vi "Laser_Setup_Options.vi"() -> (0 "Lasers IP Numbers":string[](array[string]), 1 "Wavelengths":dbl[](array[numeric]), 2 "error out":errorcluster, 3 "Lasers":string[](array[string]))   [LabVIEW 2022 SP3]
uses:
  <vilib>/Utility/error.llb/Trim Whitespace One-Sided.vi
  Globals/LDA_global.vi
  Globals/Constants_global.vi
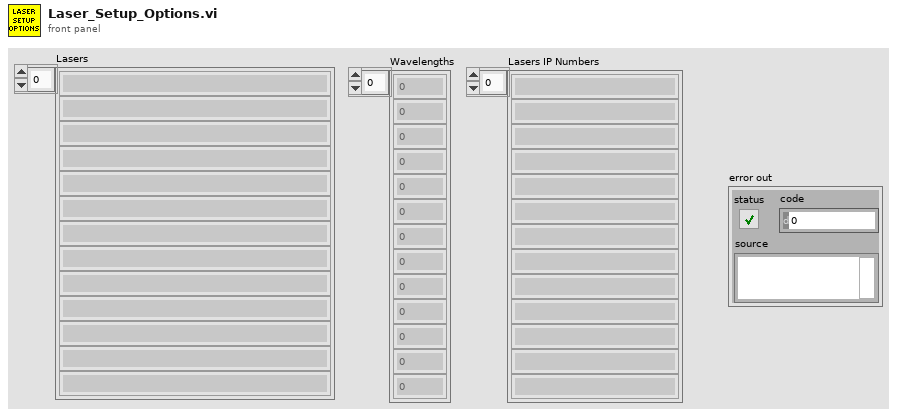
[diagram p1: front panel]
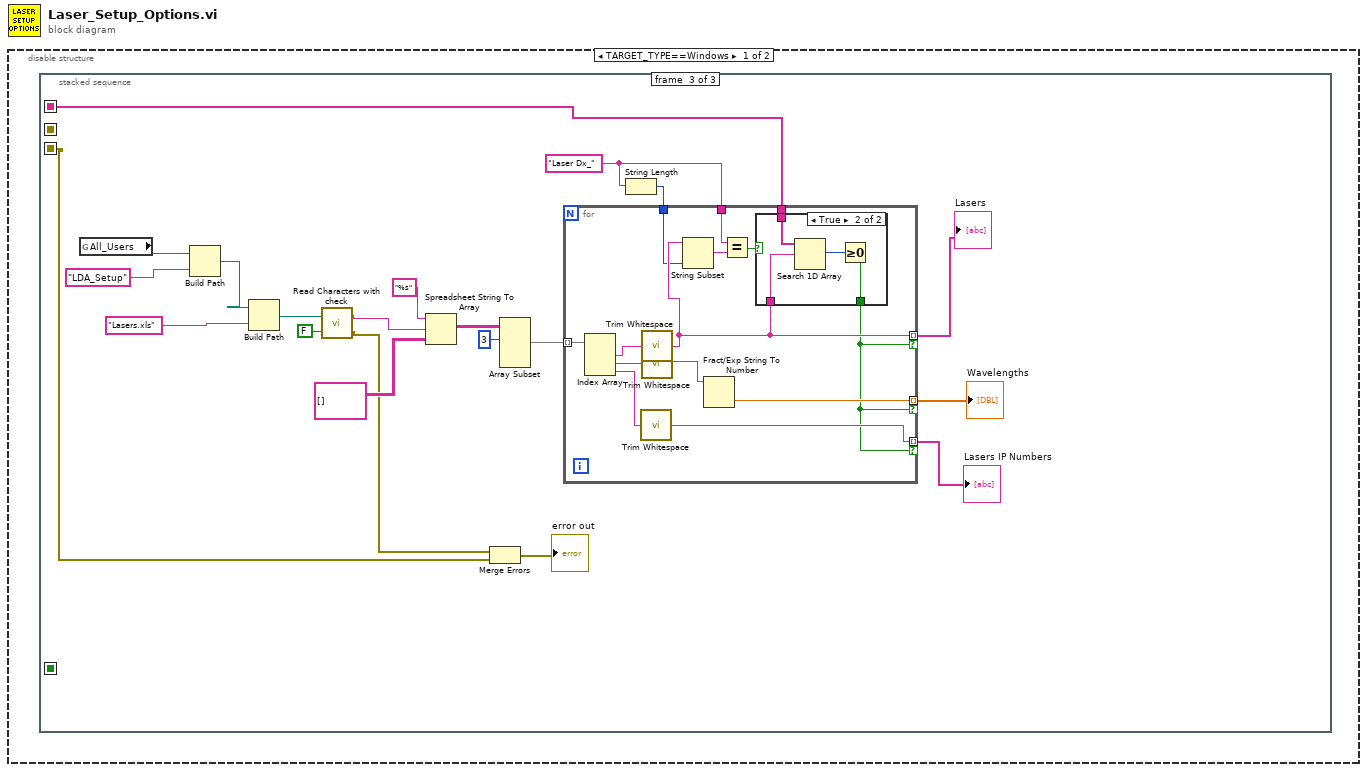
[diagram p0: block diagram]
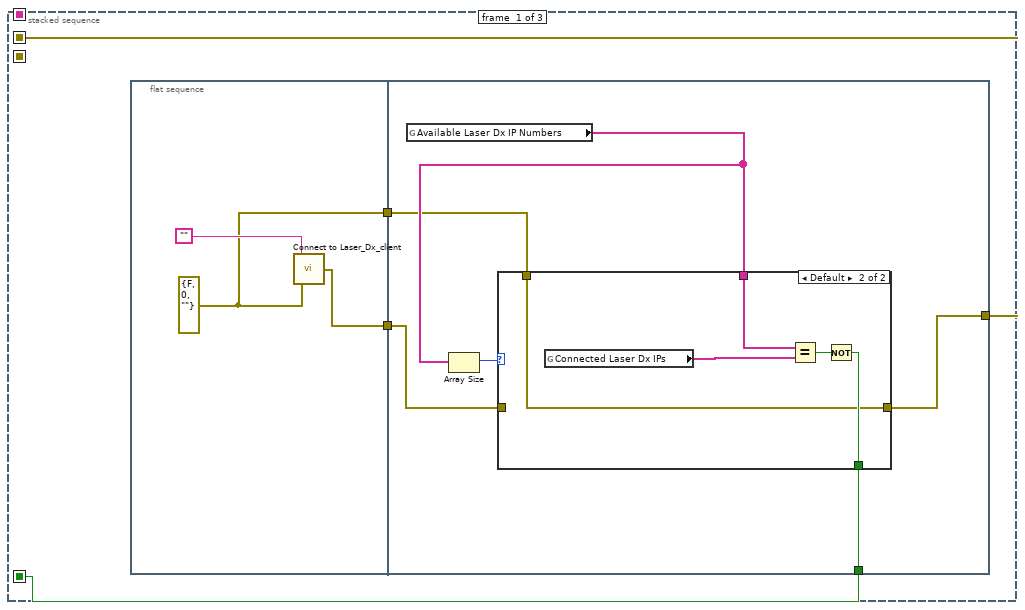
[diagram p2: hidden frame]
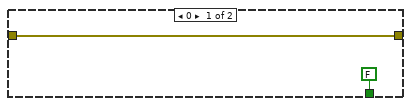
[diagram p3: hidden frame]
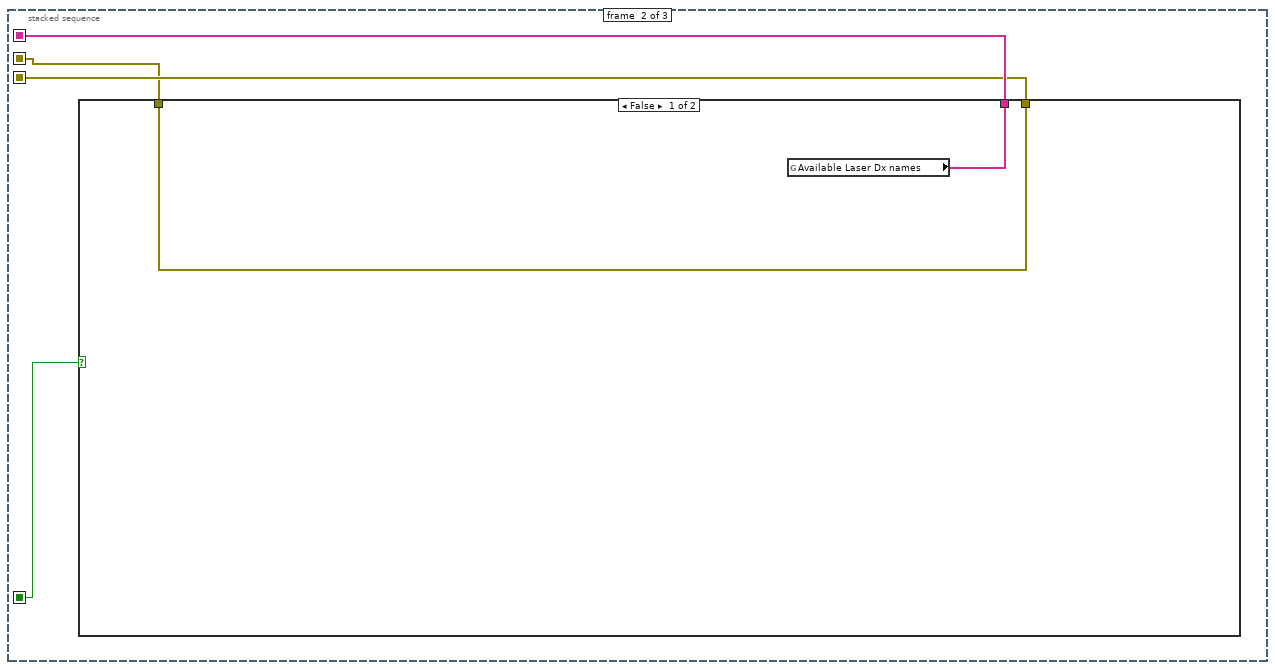
[diagram p4: hidden frame]
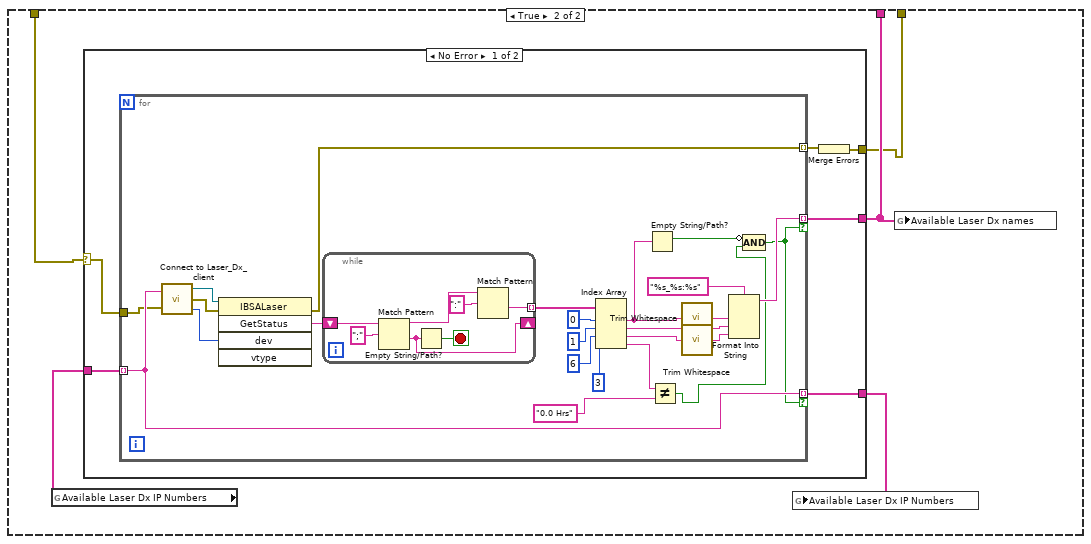
[diagram p5: hidden frame]
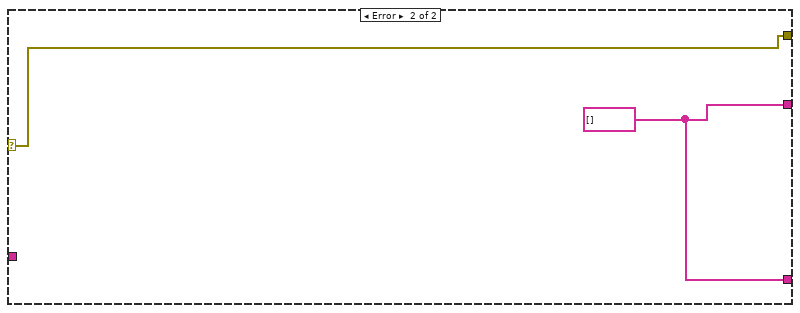
[diagram p6: hidden frame]
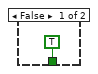
[diagram p7: hidden frame]
diagram:
  n1 = disable-structure shown="TARGET_TYPE==Windows" {
    frame condition #0 (active) {
      n2 = stacked-sequence {
        seq-local: [_ w24 _] -> [_ _ w77]
        seq-local: [_ w23 _] -> [_ _ w76]
        seq-local: [w3 _ _] -> [_ w22 _]
        seq-local: [w1 _ _] -> [_ w21 _]
        frame #0 {
          n3 = flat-sequence {
            tunnel: [w6] -> w4
            tunnel: [w5] -> w2
            tunnel: w4 -> [w10]
            tunnel: [w11] -> w3
            tunnel: w2 -> [w8]
            tunnel: [w9] -> w1
            frame #0 {
              w5 = errorcluster {"status"=FALSE, "code"=0, "source"=""} ("error in (no error)")
              n4 = call "Connect to Laser_Dx_client.vi"("Laser IP Number"="", "error in (no error)"=w5) -> ("error out"=w6:errorcluster)  [unwired: 2 out]
            }
            frame #1 {
              n5 = global read "LDA_global.vi" "Available Laser Dx IP Numbers"() -> (w13:string[])
              n6 = Array Size(array=w13) -> (size(s)=w12:i32)
              n7 = case shown="Default" w12 {
                tunnel: w13 -> [_ w19]
                tunnel: [w15 w16] -> w11
                tunnel: w10 -> [w15 _]
                tunnel: [FALSE w17] -> w9
                tunnel: w8 -> [_ w16]
                frame 0 {
                }
                frame Default {
                  n8 = global read "LDA_global.vi" "Connected Laser Dx IPs"() -> (w20:string[])
                  n9 = Equal?(x=w19, y=w20) -> (x = y?=w18:bool)
                  n10 = Not(x=w18) -> (.not. x?=w17:bool)
                }
              }
            }
          }
        }
        frame #1 {
          n11 = case shown="False" w21 {
            tunnel: [w26 w30] -> w24
            tunnel: [w25 w28] -> w23
            tunnel: w22 -> [w25 w27]
            frame False {
              n12 = global read "LDA_global.vi" "Available Laser Dx names"() -> (w26:string[])
            }
            frame True {
              n13 = global read "LDA_global.vi" "Available Laser Dx IP Numbers"() -> (w31:string[])
              n14 = case shown="No Error" w27 {
                selector: w27 -> [w32 w70]
                tunnel: w31 -> [w37 _]
                tunnel: [w36 w69] -> w30
                tunnel: [w35 w69] -> w29
                tunnel: [w33 w70] -> w28
                frame No Error {
                  n15 = for {
                    tunnel: [w51] -> w36 mode=indexing if=w38
                    tunnel: w37 -> [w46] mode=indexing
                    tunnel: [w46] -> w35 mode=indexing if=w38
                    tunnel: w32 -> [w43]
                    tunnel: [w42] -> w34 mode=indexing
                    n16 = call "Connect to Laser_Dx_client.vi"("Laser IP Number"=w46, "error in (no error)"=w43) -> ("Laser_Dx"=w50:refnum<k7>, "error out"=w45:errorcluster, "Channel"=w44:i64)
                    n17 = invoke class="IBSALaser" method="GetStatus"(reference=w50, error in=w45, "dev"=w44) -> (error out=w42:errorcluster, "GetStatus"=w52:string)  [unwired: 2 in, 3 out]
                    n18 = while {
                      shift-right: [w65] -> _
                      shift-left: w52 -> [w67]
                      tunnel: [w62] -> w58 mode=indexing
                      stop <- w66 stop-if-true
                      n19 = Match Pattern(string=w67, regular expression=";") -> (before substring=w64:string, after substring=w65:string)  [unwired: 1 in, 2 out]
                      n20 = Empty String/Path?(string/path=w65) -> (empty?=w66:bool)
                      n21 = Match Pattern(string=w64, regular expression=":") -> (after substring=w62:string)  [unwired: 1 in, 3 out]
                    }
                    n22 = Index Array(array=w58, index #1=0 ("index"), index #2=1 ("index"), index #3=6 ("index"), index #4=3 ("index")) -> (element #1=w41:string, element #2=w56:string, element #3=w59:string, element #4=w47:string)
                    n23 = Empty String/Path?(string/path=w41) -> (empty?=w40:bool)
                    n24 = Not Equal?(x=w47, y="0.0 Hrs" ("element")) -> (x != y?=w39:bool)
                    n25 = call <vilib>:"Trim Whitespace.vi"("string"=w41) -> ("trimmed string"=w61:string)  [unwired: 1 in]
                    n26 = call <vilib>:"Trim Whitespace.vi"("string"=w59) -> ("trimmed string"=w60:string)  [unwired: 1 in]
                    n27 = Format Into String(format string="%s_%s:%s", w61, w56, w60) -> (resulting string=w51:string)  [unwired: 2 in, 1 out]
                    n28 = Compound Arithmetic op=AND(invert w40, w39) -> (w38:bool)
                  }
                  n29 = Merge Errors(w34) -> (w33:errorcluster)
                }
                frame Error {
                  w69 = string[] []
                }
              }
              n30 = global write "LDA_global.vi" "Available Laser Dx IP Numbers"(w29) -> ()
              n31 = global write "LDA_global.vi" "Available Laser Dx names"(w30) -> ()
            }
          }
        }
        frame #2 {
          w79 = "Laser Dx_"
          n32 = global read "Constants_global.vi" "All_Users"() -> (w89:path)
          n33 = Build Path(base path=w89, name or relative path="LDA_Setup") -> (appended path=w88:path)
          n34 = Build Path(base path=w88, name or relative path="Lasers.xls") -> (appended path=w74:path)
          n35 = call "Read Characters with check.vi"("Call EnFlo Error Handler?"=FALSE, "file (use dialog)"=w74) -> ("error out"=w72:errorcluster, "Read String"=w73:string)
          n36 = Spreadsheet String To Array(format string="%s", spreadsheet string=w73, array type (2D Dbl)=string[][] []) -> (array=w85:string[][])  [unwired: 1 in]
          n37 = Merge Errors(w72, w76) -> (→"error out":errorcluster)
          n38 = Array Subset(array=w85, index (row)=3 ("index")) -> (w81:string[][])  [unwired: 3 in]
          n39 = String Length(string=w79) -> (length=w80:i32)
          n40 = for {
            tunnel: w81 -> [w105] mode=indexing
            tunnel: [w99] -> w91 mode=indexing if=w92
            tunnel: [w101] -> w90 mode=indexing if=w92
            tunnel: w77 -> [w100]
            tunnel: w80 -> [w98]
            tunnel: w79 -> [w96]
            tunnel: [w93] -> w78 mode=indexing if=w92
            n41 = Index Array(array=w105) -> (element #1=w104:string, element #2=w103:string, element #3=w94:string)  [unwired: 3 in]
            n42 = call <vilib>:"Trim Whitespace.vi"("string"=w94) -> ("trimmed string"=w93:string)  [unwired: 1 in]
            n43 = call <vilib>:"Trim Whitespace.vi"("string"=w104) -> ("trimmed string"=w99:string)  [unwired: 1 in]
            n44 = call <vilib>:"Trim Whitespace.vi"("string"=w103) -> ("trimmed string"=w102:string)  [unwired: 1 in]
            n45 = String Subset(string=w99, length (rest)=w98) -> (substring=w97:string)  [unwired: 1 in]
            n46 = Fract/Exp String To Number(string=w102) -> (number=w101:dbl)  [unwired: 3 in, 1 out]
            n47 = Equal?(x=w96, y=w97) -> (x = y?=w95:bool)
            n48 = case shown="True" w95 {
              tunnel: w100 -> [_ w110]
              tunnel: w99 -> [_ w109]
              tunnel: [TRUE w107] -> w92
              frame False {
              }
              frame True {
                n49 = Search 1D Array(1D array=w110, element=w109) -> (index of element=w108:i32)  [unwired: 1 in]
                n50 = Greater Or Equal To 0?(x=w108) -> (x >= 0?=w107:bool)
              }
            }
          }
          "Wavelengths" <- w90
          "Lasers" <- w91
          "Lasers IP Numbers" <- w78
        }
      }
    }
    frame condition #1 {
    }
  }
